vi "FormProductsTable.vi"() -> ()   [LabVIEW 2012]
uses:
  resultShow.vi
  S7Ref.vi
panel:
  in  "检具选择":bool[](array[boolean])
  in  "判定设定 2":string[][](table)
  in  "参数设定 2":string[][](table)
  in  "判定设定":string[][](table)
  in  "参数设定":string[][](table)
  in  "产品选择":bool
  in  "产品删除":bool
  in  "产品更新":bool
  in  "产品注册":bool
  in  "产品":string(combo)
  # "检具15"
  # "检具1"
  # "检具2"
  # "检具3"
  # "检具4"
  # "检具5"
  # "检具6"
  # "检具7"
  # "检具8"
  # "检具9"
  # "检具10"
  # "检具11"
  # "检具12"
  # "检具13"
  # "检具14"
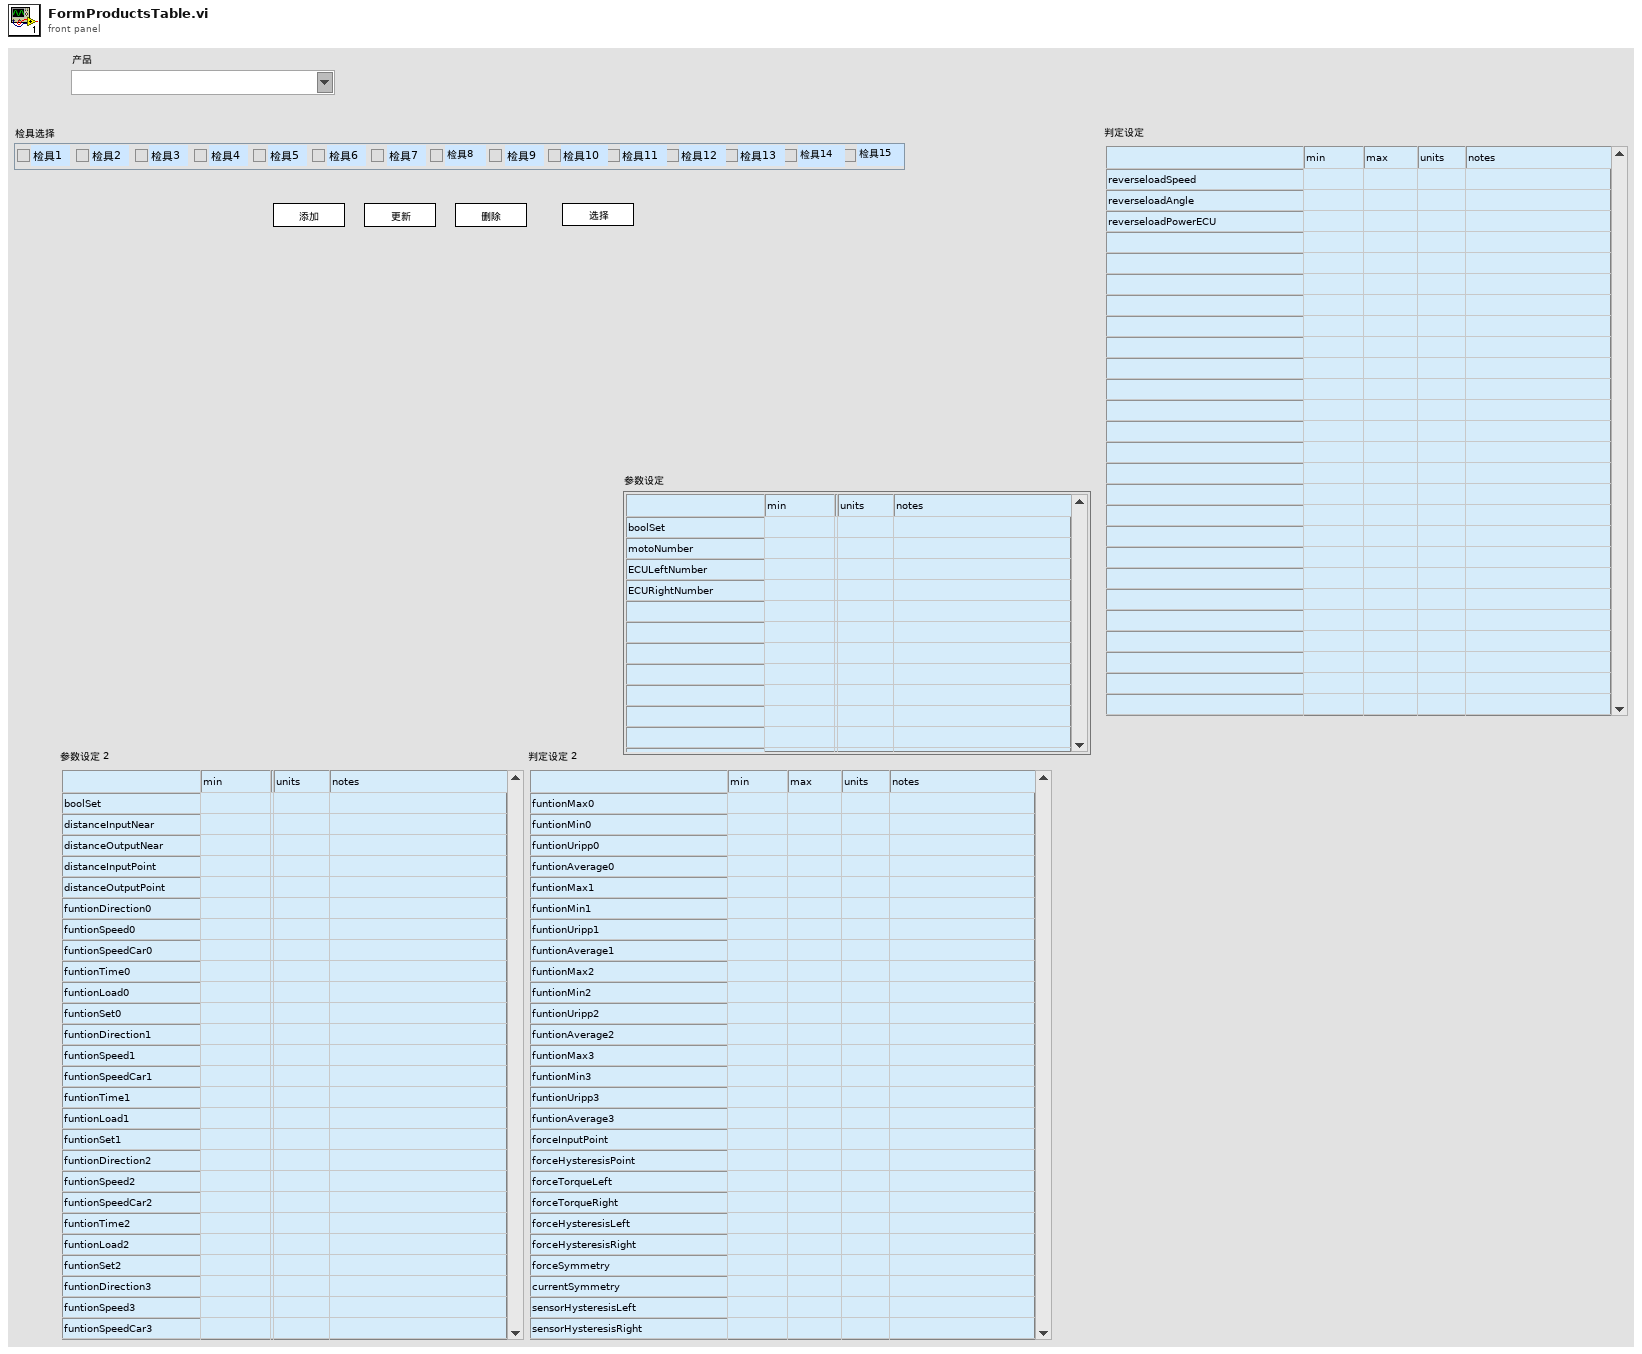
[diagram p1: front panel]
types:
  T1 = enum8{"Enabled", "Disabled", "Disabled and Grayed Out"}
  T2 = enum16{"selectdata", "selectsave", "selectlist", "selectshow"}
  T3 = cluster{"userCode":string, "userName":string, "userStatus":string, "connectionMode":string, "takesTime":string, "countDone":string, "countOK":string, "countNG":string, "rigStatus":string, "productsName":string, "partCode1":string, "partCode2":string, "partCode3":string}
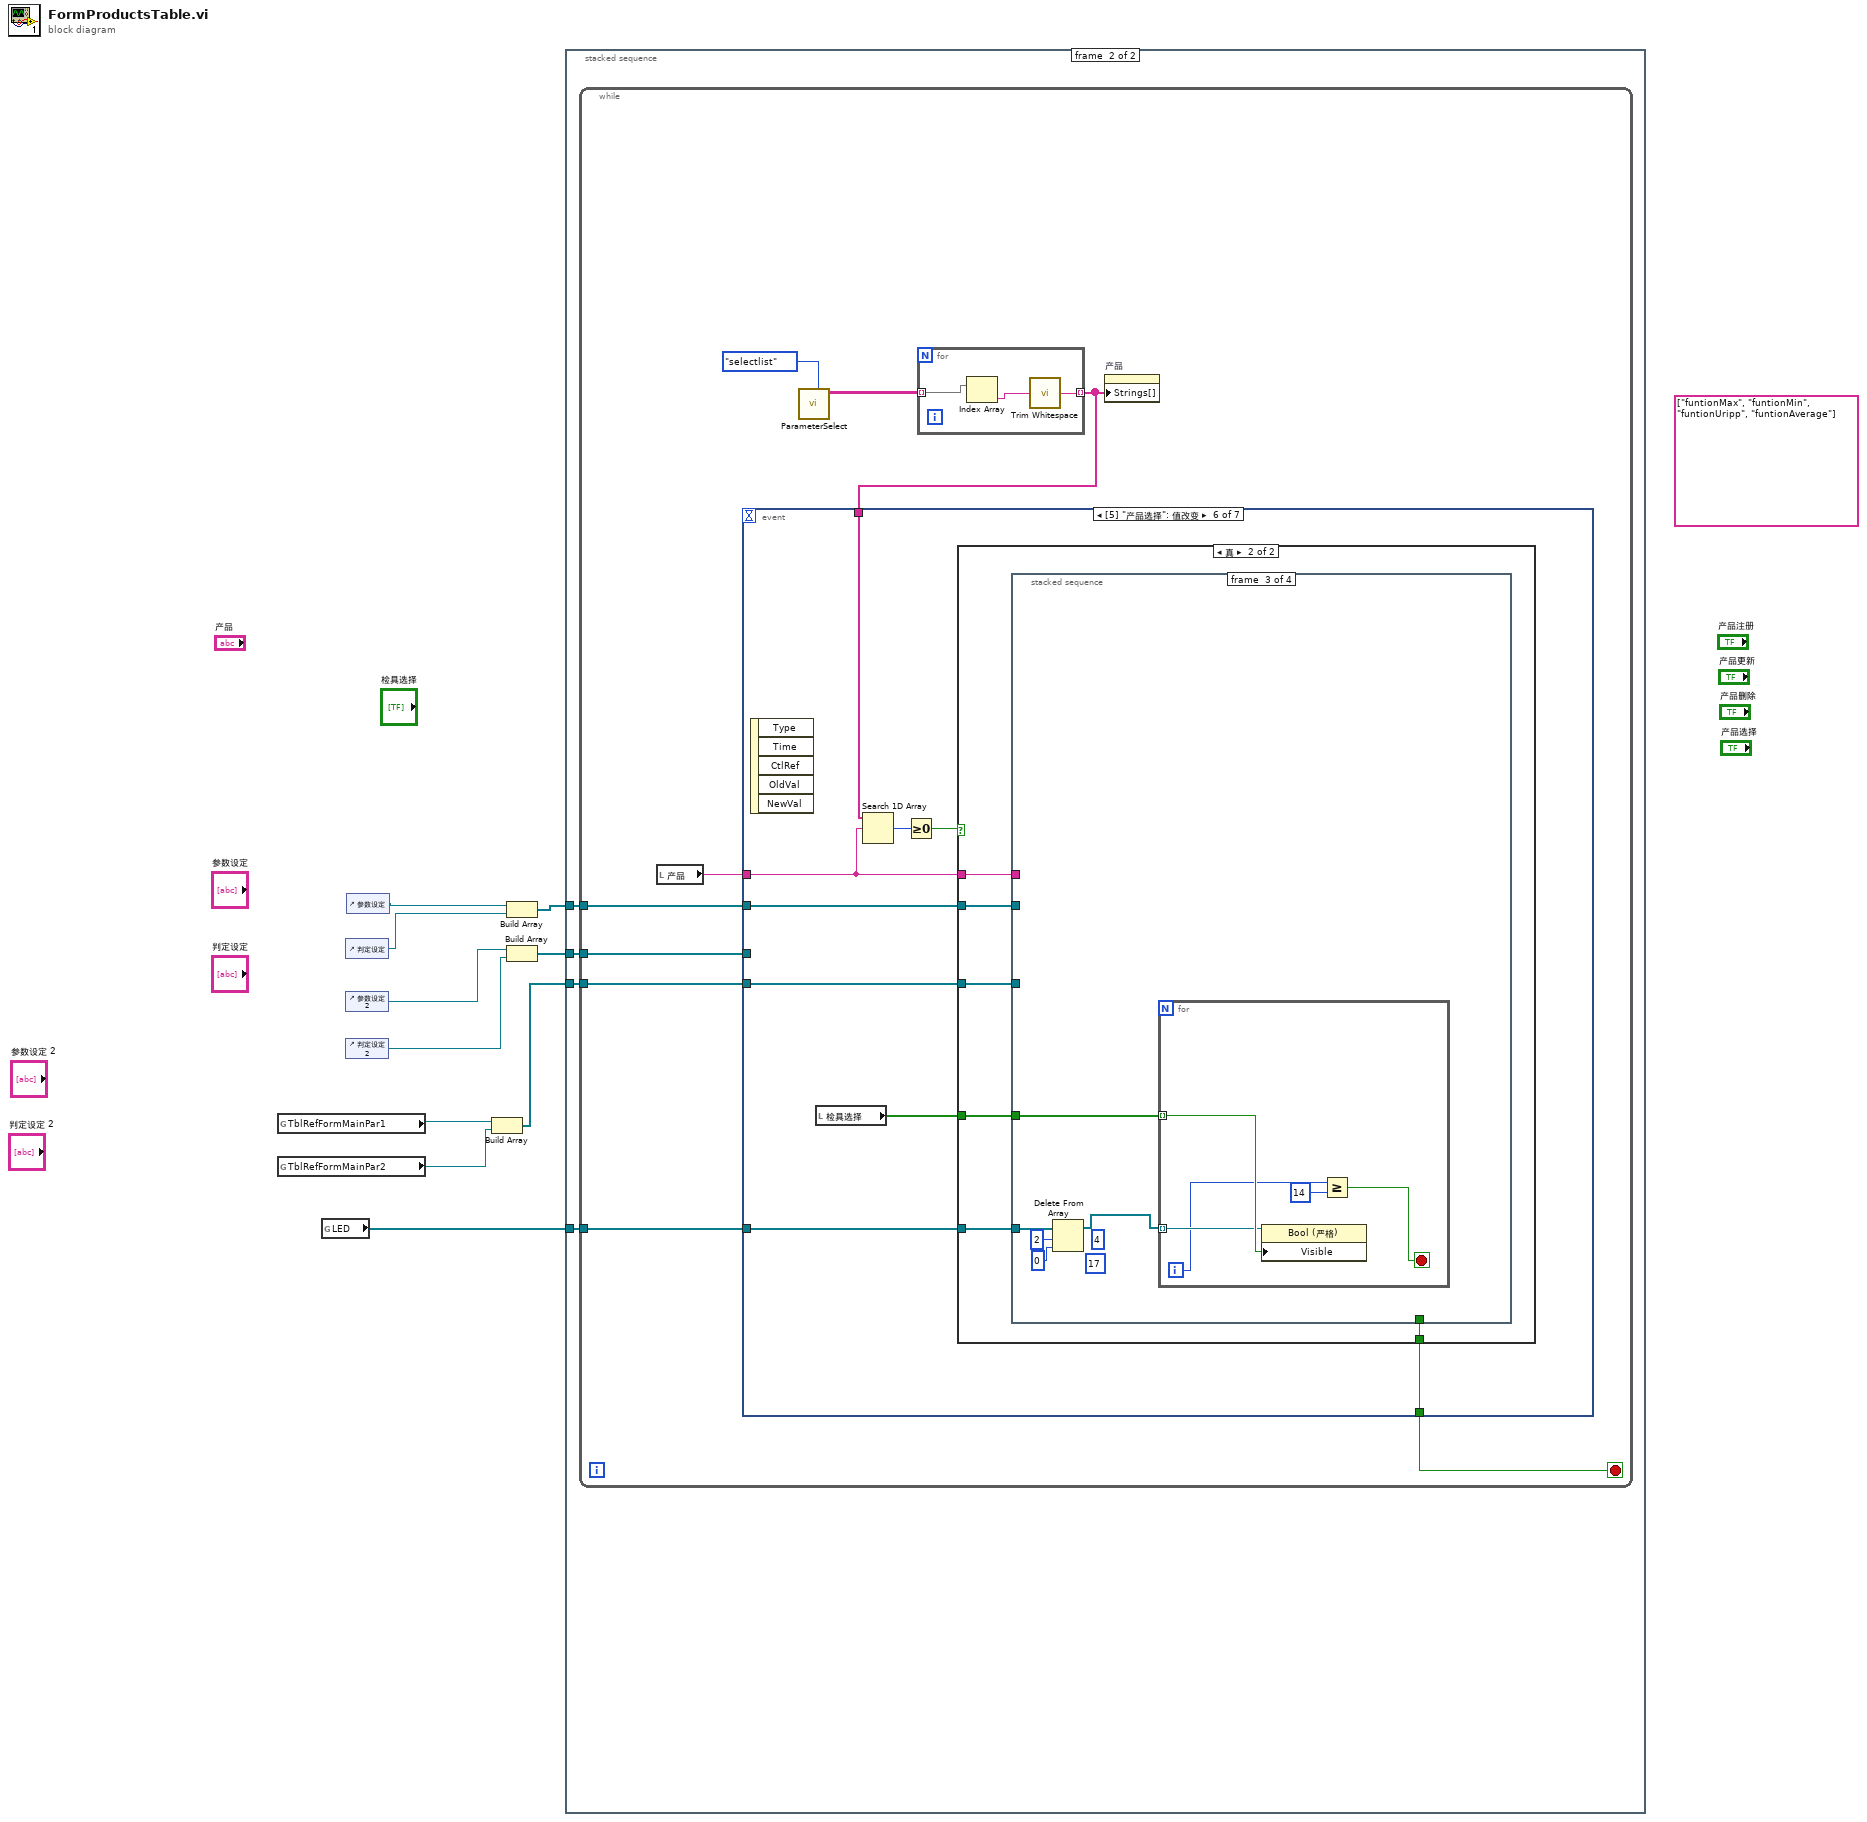
[diagram p0: block diagram]
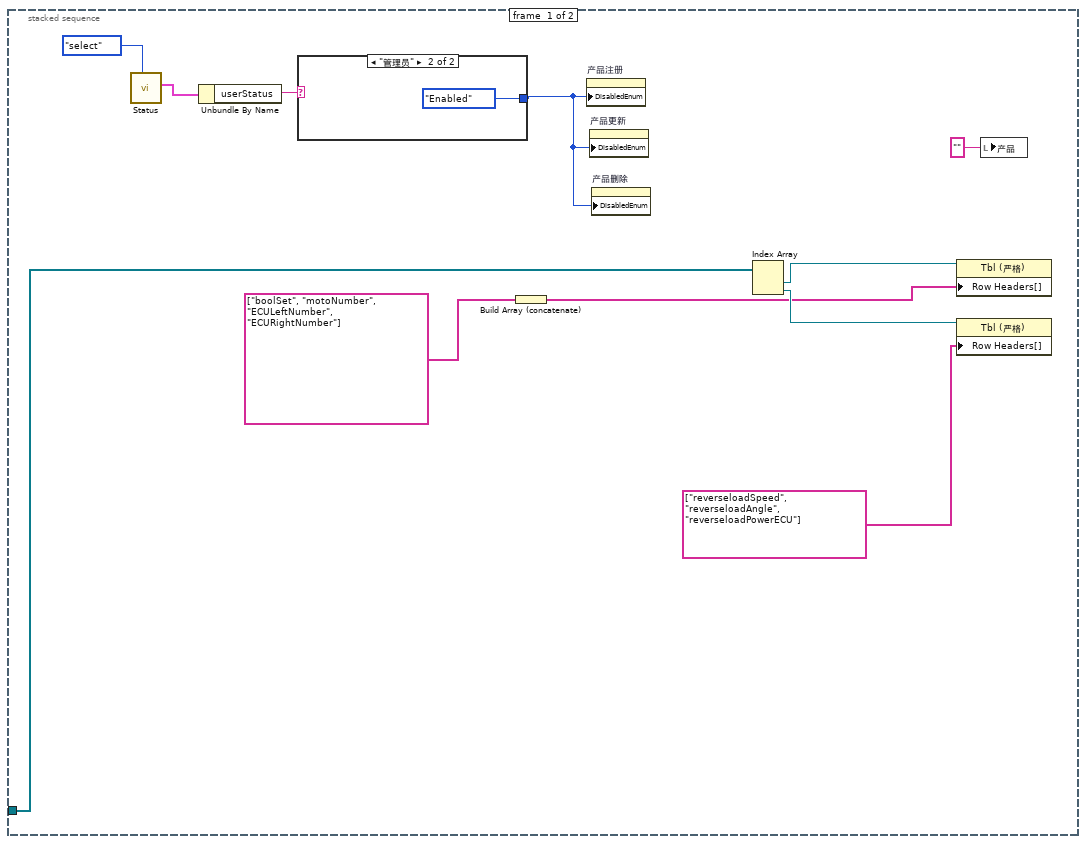
[diagram p2: hidden frame]
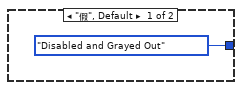
[diagram p3: hidden frame]
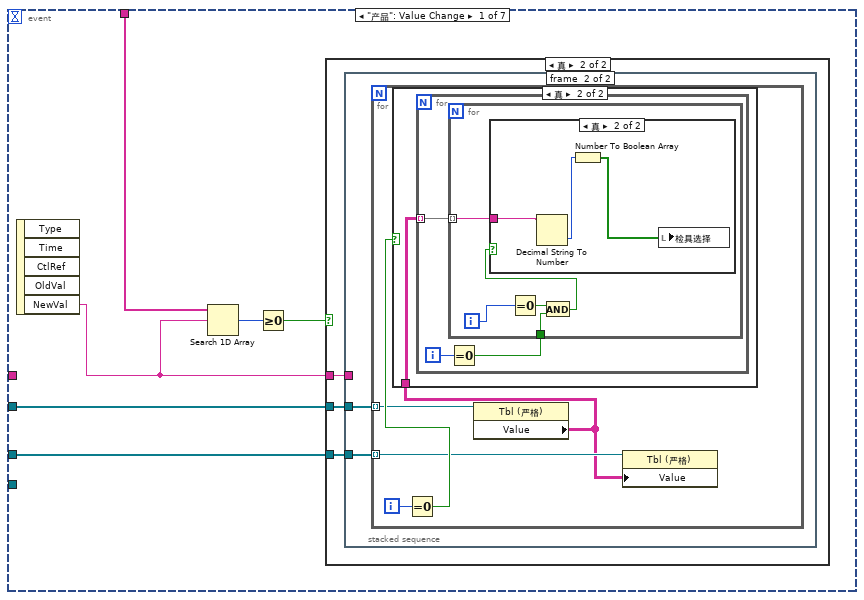
[diagram p4: hidden frame]
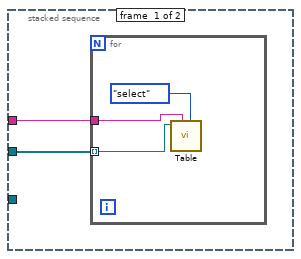
[diagram p6: hidden frame]
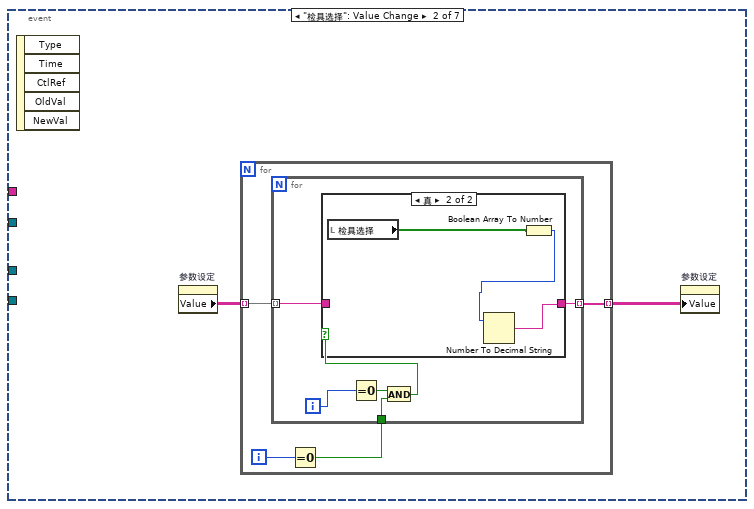
[diagram p9: hidden frame]
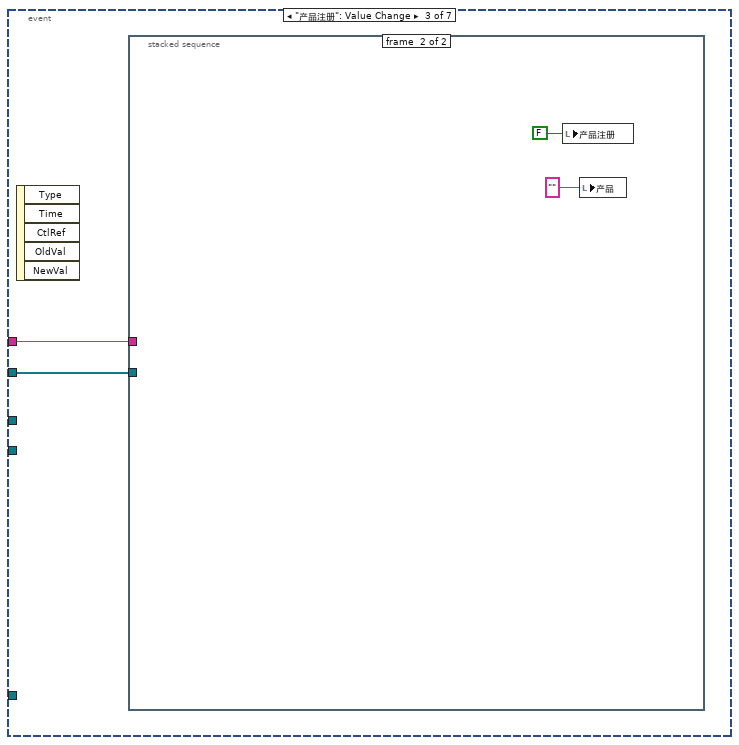
[diagram p11: hidden frame]
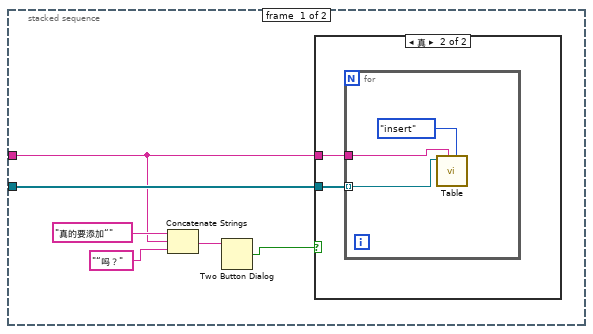
[diagram p12: hidden frame]
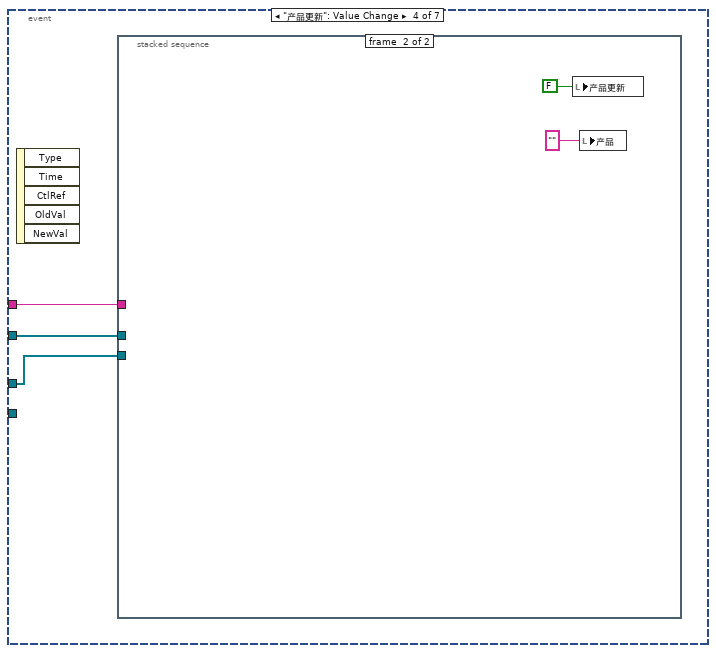
[diagram p14: hidden frame]
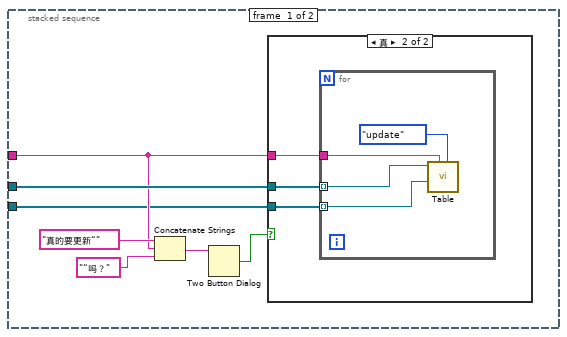
[diagram p15: hidden frame]
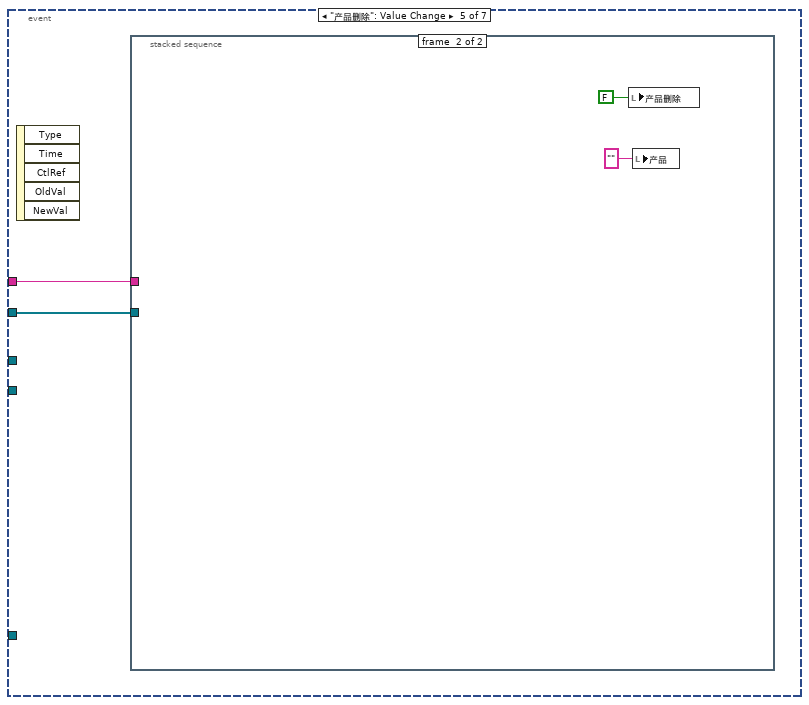
[diagram p17: hidden frame]
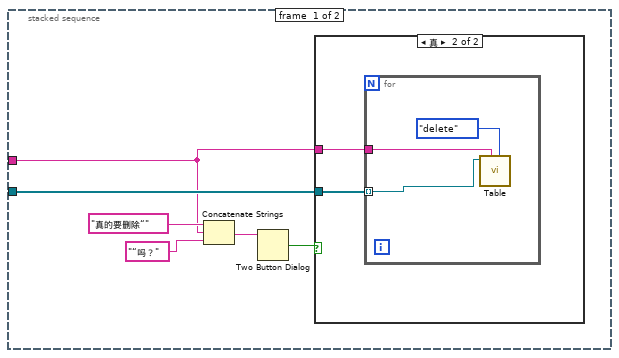
[diagram p18: hidden frame]
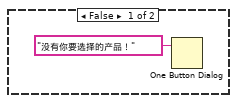
[diagram p20: hidden frame]
diagram:
  (unwired) string[] ["funtionMax", "funtionMin", "funtionUripp", "funtionAverage"] ("字符串[]")
  n1 = global read "resultShow.vi" "TblRefFormMainPar1"() -> (w6:refnum<vi>)
  n2 = global read "resultShow.vi" "TblRefFormMainPar2"() -> (w5:refnum<vi>)
  n3 = global read "resultShow.vi" "LED"() -> (w1:refnum<vi>[])
  n4 = control-ref of="判定设定"() -> (w8:refnum<vi>)
  n5 = control-ref of="参数设定 2"() -> (w3:refnum<vi>)
  n6 = control-ref of="判定设定 2"() -> (w4:refnum<vi>)
  n7 = control-ref of="参数设定"() -> (w9:refnum<vi>)
  n8 = Build Array(w6, w5) -> (w7:refnum<vi>[])
  n9 = Build Array(w9, w8) -> (w10:refnum<vi>[])
  n10 = Build Array(w3, w4) -> (w2:refnum<vi>[])
  n11 = stacked-sequence {
    tunnel: w10 -> [w14 w27]
    tunnel: w7 -> [_ w26]
    tunnel: w2 -> [_ w25]
    tunnel: w1 -> [_ w24]
    frame #0 {
      n12 = call "Status.vi"("模式"=enum16{"select", "insert", "update", "delete"}."select") -> ("元素"=w18:T3)  [unwired: 10 in]
      n13 = Unbundle By Name(w18) -> ("userStatus"=w20:string)
      n14 = case shown="\"管理员\"" w20 {
        tunnel: [T1."Disabled and Grayed Out" ("禁用") T1."Enabled" ("禁用")] -> w17
        frame "假", Default {
        }
        frame "管理员" {
        }
      }
      n15 = Build Array (concatenate)(string[] ["boolSet", "motoNumber", "ECULeftNumber", "ECURightNumber"] ("字符串[]")) -> (w13:string[])
      n16 = property on="产品注册" class="Bool (严格)"("DisabledEnum"=w17) -> ()  [unwired: 2 in, 2 out]
      n17 = property on="产品更新" class="Bool (严格)"("DisabledEnum"=w17) -> ()  [unwired: 2 in, 2 out]
      n18 = property on="产品删除" class="Bool (严格)"("DisabledEnum"=w17) -> ()  [unwired: 2 in, 2 out]
      n19 = Index Array(array=w14) -> (element #1=w16:refnum<vi>, element #2=w15:refnum<vi>)  [unwired: 2 in]
      n20 = property class="Tbl (严格)"(reference=w16, "Row Headers[]"=w13) -> ()  [unwired: 1 in, 2 out]
      n21 = property class="Tbl (严格)"(reference=w15, "Row Headers[]"=string[] ["reverseloadSpeed", "reverseloadAngle", "reverseloadPowerECU"] ("字符串[]")) -> ()  [unwired: 1 in, 2 out]
      n22 = local write "产品"("" ("y")) -> ()
    }
    frame #1 {
      n23 = while {
        tunnel: w27 -> [w33]
        tunnel: w26 -> [w30]
        tunnel: w25 -> [w29]
        tunnel: w24 -> [w28]
        stop <- w36 stop-if-true
        n24 = local read "产品"() -> (w35:string)
        n25 = call "ParameterSelect.vi"("模式"=T2."selectlist") -> ("dataOutAll"=w32:string[][])  [unwired: 5 in, 5 out]
        n26 = for {
          tunnel: w32 -> [w38] mode=indexing
          tunnel: [w39] -> w34 mode=indexing
          n27 = Index Array(array=w38) -> (element=w37:string)  [unwired: 1 in]
          n28 = call <vilib>:"Trim Whitespace.vi"("string"=w37) -> ("trimmed string"=w39:string)  [unwired: 1 in]
        }
        n29 = event shown="[5] \"产品选择\": 值改变" {
          selector: _ -> [_ _ _ _ _ _ _]
          dyn-events: _ -> [_ _ _ _ _ _ _]
          timeout: _ -> [_ _ _ _ _ _ _]
          tunnel: [_ _ _ _ _ w146 w204] -> w36
          tunnel: w33 -> [w45 _ w90 w106 w124 w141 _]
          tunnel: w35 -> [_ _ w89 w105 w123 w144 _]
          tunnel: w34 -> [w44 _ _ _ _ w145 _]
          tunnel: w30 -> [_ _ _ _ _ w140 _]
          tunnel: w29 -> [w40 _ _ w104 _ _ _]
          tunnel: w28 -> [_ _ _ _ _ w139 _]
          event "产品": Value Change {
            n30 = event-data() -> ("NewVal"=w42:string)  [unwired: 1 in, 4 out]
            n31 = Search 1D Array(1D array=w44, element=w42) -> (index of element=w43:i32)  [unwired: 1 in]
            n32 = Greater Or Equal To 0?(x=w43) -> (x >= 0?=w41:bool)
            n33 = case shown="真" w41 {
              tunnel: w45 -> [_ w48]
              tunnel: w42 -> [_ w47]
              tunnel: w40 -> [_ w46]
              frame False {
              }
              frame True {
                n34 = stacked-sequence {
                  tunnel: w48 -> [w50 w55]
                  tunnel: w47 -> [w49 _]
                  tunnel: w46 -> [_ w54]
                  frame #0 {
                    n35 = for {
                      tunnel: w50 -> [w53] mode=indexing
                      tunnel: w49 -> [w52]
                      n36 = call "Table.vi"("模式"=enum16{"select", "insert", "update", "delete"}."select", "productsName"=w52, "Table"=w53) -> ()  [unwired: 9 in]
                    }
                  }
                  frame #1 {
                    n37 = for {
                      tunnel: w55 -> [w58] mode=indexing
                      tunnel: w54 -> [w57] mode=indexing
                      i -> [w59]
                      n38 = Equal To 0?(x=w59) -> (x = 0?=w60:bool)
                      n39 = property on="属性节点" class="Tbl (严格)"(reference=w58) -> ("Value"=w56:string[][])  [unwired: 1 in, 2 out]
                      n40 = case shown="真" w60 {
                        tunnel: w56 -> [_ w61]
                        frame False {
                        }
                        frame True {
                          n41 = for {
                            tunnel: w61 -> [w62] mode=indexing
                            i -> [w64]
                            n42 = Equal To 0?(x=w64) -> (x = 0?=w63:bool)
                            n43 = for {
                              tunnel: w62 -> [w66] mode=indexing
                              tunnel: w63 -> [w67]
                              i -> [w68]
                              n44 = Equal To 0?(x=w68) -> (x = 0?=w69:bool)
                              n45 = And(x=w69, y=w67) -> (x .and. y?=w65:bool)
                              n46 = case shown="真" w65 {
                                tunnel: w66 -> [_ w72]
                                frame False {
                                }
                                frame True {
                                n47 = Decimal String To Number(string=w72) -> (number=w71:i32)  [unwired: 2 in, 1 out]
                                n48 = Number To Boolean Array(number=w71) -> (Boolean array=w70:bool[])
                                n49 = local write "检具选择"(w70) -> ()
                                }
                              }
                            }
                          }
                        }
                      }
                      n50 = property on="属性节点" class="Tbl (严格)"(reference=w57, "Value"=w56) -> ()  [unwired: 1 in, 2 out]
                    }
                  }
                }
              }
            }
          }
          event "检具选择": Value Change {
            n51 = event-data() -> ()  [unwired: 1 in, 5 out]
            n52 = property on="参数设定" class="Tbl (严格)"() -> ("Value"=w74:string[][])  [unwired: 2 in, 2 out]
            n53 = for {
              tunnel: w74 -> [w78] mode=indexing
              tunnel: [w75] -> w73 mode=indexing
              i -> [w77]
              n54 = Equal To 0?(x=w77) -> (x = 0?=w76:bool)
              n55 = for {
                tunnel: w78 -> [w80] mode=indexing
                tunnel: w76 -> [w82]
                tunnel: [w81] -> w75 mode=indexing
                i -> [w83]
                n56 = Equal To 0?(x=w83) -> (x = 0?=w84:bool)
                n57 = And(x=w84, y=w82) -> (x .and. y?=w79:bool)
                n58 = case shown="真" w79 {
                  tunnel: [w85 w87] -> w81
                  tunnel: w80 -> [w85 _]
                  frame False {
                  }
                  frame True {
                    n59 = local read "检具选择"() -> (w86:bool[])
                    n60 = Boolean Array To Number(Boolean array=w86) -> (number=w88:u32)
                    n61 = Number To Decimal String(number=w88) -> (decimal integer string=w87:string)  [unwired: 1 in]
                  }
                }
              }
            }
            n62 = property on="参数设定" class="Tbl (严格)"("Value"=w73) -> ()  [unwired: 2 in, 2 out]
          }
          event "产品注册": Value Change {
            n63 = event-data() -> ()  [unwired: 1 in, 5 out]
            n64 = stacked-sequence {
              tunnel: w90 -> [w96 _]
              tunnel: w89 -> [w91 _]
              frame #0 {
                n65 = Concatenate Strings("真的要添加“" ("消息"), w91, "“吗？" ("消息")) -> (w93:string)
                n66 = Two Button Dialog(message=w93) -> (T button?=w92:bool)  [unwired: 2 in]
                n67 = case shown="真" w92 {
                  tunnel: w96 -> [_ w98]
                  tunnel: w91 -> [_ w97]
                  frame False {
                  }
                  frame True {
                    n68 = for {
                      tunnel: w98 -> [w100] mode=indexing
                      tunnel: w97 -> [w99]
                      n69 = call "Table.vi"("模式"=enum16{"select", "insert", "update", "delete"}."insert", "productsName"=w99, "Table"=w100) -> ()  [unwired: 9 in]
                    }
                  }
                }
              }
              frame #1 {
                n70 = local write "产品注册"(FALSE ("产品注册")) -> ()
                n71 = local write "产品"("") -> ()
              }
            }
          }
          event "产品更新": Value Change {
            n72 = event-data() -> ()  [unwired: 1 in, 5 out]
            n73 = stacked-sequence {
              tunnel: w106 -> [w113 _]
              tunnel: w105 -> [w108 _]
              tunnel: w104 -> [w107 _]
              frame #0 {
                n74 = Concatenate Strings("真的要更新“" ("消息"), w108, "“吗？" ("消息")) -> (w110:string)
                n75 = Two Button Dialog(message=w110) -> (T button?=w109:bool)  [unwired: 2 in]
                n76 = case shown="真" w109 {
                  tunnel: w113 -> [_ w116]
                  tunnel: w108 -> [_ w115]
                  tunnel: w107 -> [_ w114]
                  frame False {
                  }
                  frame True {
                    n77 = for {
                      tunnel: w116 -> [w119] mode=indexing
                      tunnel: w115 -> [w118]
                      tunnel: w114 -> [w117] mode=indexing
                      n78 = call "Table.vi"("模式"=enum16{"select", "insert", "update", "delete"}."update", "productsName"=w118, "Table 2"=w117, "Table"=w119) -> ()  [unwired: 8 in]
                    }
                  }
                }
              }
              frame #1 {
                n79 = local write "产品更新"(FALSE ("产品注册")) -> ()
                n80 = local write "产品"("") -> ()
              }
            }
          }
          event "产品删除": Value Change {
            n81 = event-data() -> ()  [unwired: 1 in, 5 out]
            n82 = stacked-sequence {
              tunnel: w124 -> [w130 _]
              tunnel: w123 -> [w125 _]
              frame #0 {
                n83 = Concatenate Strings("真的要删除“" ("消息"), w125, "“吗？" ("消息")) -> (w127:string)
                n84 = Two Button Dialog(message=w127) -> (T button?=w126:bool)  [unwired: 2 in]
                n85 = case shown="真" w126 {
                  tunnel: w130 -> [_ w132]
                  tunnel: w125 -> [_ w131]
                  frame False {
                  }
                  frame True {
                    n86 = for {
                      tunnel: w132 -> [w134] mode=indexing
                      tunnel: w131 -> [w133]
                      n87 = call "Table.vi"("模式"=enum16{"select", "insert", "update", "delete"}."delete", "productsName"=w133, "Table"=w134) -> ()  [unwired: 9 in]
                    }
                  }
                }
              }
              frame #1 {
                n88 = local write "产品删除"(FALSE ("产品删除")) -> ()
                n89 = local write "产品"("" ("products_name_in")) -> ()
              }
            }
          }
          event "产品选择": Value Change {
            n90 = event-data() -> ()  [unwired: 1 in, 5 out]
            n91 = local read "检具选择"() -> (w138:bool[])
            n92 = Search 1D Array(1D array=w145, element=w144) -> (index of element=w143:i32)  [unwired: 1 in]
            n93 = Greater Or Equal To 0?(x=w143) -> (x >= 0?=w142:bool)
            n94 = case shown="真" w142 {
              tunnel: [_ w153] -> w146
              tunnel: w144 -> [_ w152]
              tunnel: w141 -> [_ w151]
              tunnel: w140 -> [_ w150]
              tunnel: w139 -> [_ w149]
              tunnel: w138 -> [_ w148]
              frame False {
                n95 = One Button Dialog(message="没有你要选择的产品！" ("消息")) -> ()  [unwired: 1 in, 1 out]
              }
              frame True {
                n96 = stacked-sequence {
                  tunnel: w152 -> [w163 _ _ _]
                  tunnel: [_ _ _ TRUE ("产品删除")] -> w153
                  tunnel: w151 -> [w156 _ _ _]
                  tunnel: w150 -> [w157 _ _ _]
                  tunnel: w149 -> [_ w185 w191 _]
                  tunnel: w148 -> [_ _ w192 _]
                  frame #0 {
                    n97 = for {
                      tunnel: w157 -> [w167] mode=indexing
                      tunnel: w156 -> [w168] mode=indexing
                      tunnel: [w166] -> w155 mode=indexing
                      n98 = property on="属性节点" class="Tbl (严格)"(reference=w168) -> (reference out=w170:refnum<vi>, "Value"=w166:string[][])  [unwired: 1 in, 1 out]
                      n99 = property on="属性节点" class="Tbl (严格)"(reference=w170) -> ("Row Headers[]"=w169:string[])  [unwired: 1 in, 2 out]
                      n100 = property on="属性节点" class="Tbl"(reference=w167, "Value"=w166) -> (reference out=w171:refnum<vi>)  [unwired: 1 in, 1 out]
                      n101 = property on="属性节点" class="Tbl"(reference=w171, "Row Headers[]"=w169) -> ()  [unwired: 1 in, 2 out]
                    }
                    n102 = Bundle("name"="productsName", "产品"=w163) -> (w162:cluster{"name":string, "产品":string})  [unwired: 1 in]
                    n103 = Index Array(array=w155) -> (element=w154:string[][])  [unwired: 3 in]
                    n104 = Build Array(w162) -> (w161:cluster{"name":string, "产品":string}[])
                    n105 = Transpose 2D Array(2D array=w154) -> (transposed array=w158:string[][])
                    n106 = call "Status.vi"("模式"=enum16{"select", "insert", "update", "delete"}."update", "nameData"=w161) -> ()  [unwired: 9 in, 1 out]
                    n107 = Index Array(array=w158) -> (element=w160:string[])  [unwired: 2 in]
                    n108 = Fract/Exp String To Number(string=w160) -> (number=w159:dbl[])  [unwired: 3 in, 1 out]
                    n109 = for {
                      tunnel: w159 -> [w172] mode=indexing
                      i -> [w176]
                      w183 = u16 2 items=["byte", "word", "Dword"]  # 数据类型
                      (unwired) u32 1  # 写入地址
                      w182 = u16 100  # DB #
                      w184 = u8 132 items=["I/O (P)"=128, "Input (I)"=129, "Output (Q)"=130, "Bit Memory (M)"=131, "Data (DB)"=132, "Instance Data (DI)"=133, "Local Data (L)"=134, "Predecessor Local Data (VL)"=135]  # 寄存器类型
                      n110 = global read "S7Ref.vi" "S7Ref"() -> (w178:refnum<k5>)
                      n111 = Add(x=20 ("y"), y=w176) -> (x+y=w175:i32)
                      n112 = To Single Precision Float(number=w172) -> (single precision float=w173:sgl)
                      n113 = Multiply(x=w175, y=4) -> (x*y=w180:i32)
                      n114 = Type Cast(type=u32 0, x=w173) -> (*(type *) &x=w179:u32)
                      n115 = call "S7_Write.vi"("TCP"=w178, "寄存器类型"=w184, "DB #"=w182, "写入地址"=w180, "数据类型"=w183, "写入数据"=w179) -> ()  [unwired: 7 in, 3 out]
                    }
                  }
                  frame #1 {
                    n116 = for {
                      tunnel: w185 -> [w187] mode=indexing
                      n117 = property class="Bool (严格)"(reference=w187, "Visible"=TRUE ("可见")) -> ()  [unwired: 1 in, 2 out]
                    }
                  }
                  frame #2 {
                    (unwired) 17 ("索引")
                    (unwired) 4 ("长度")
                    n118 = Delete From Array(array=w191, length=2 ("长度"), index=0 ("索引")) -> (array with subset deleted=w188:refnum<vi>[])  [unwired: 1 out]
                    n119 = for {
                      tunnel: w188 -> [w196] mode=indexing
                      tunnel: w192 -> [w197] mode=indexing
                      i -> [w195]
                      stop <- w193 stop-if-true
                      n120 = property class="Bool (严格)"(reference=w196, "Visible"=w197) -> ()  [unwired: 1 in, 2 out]
                      n121 = Greater Or Equal?(x=w195, y=14) -> (x >= y?=w193:bool)
                    }
                  }
                  frame #3 {
                    n122 = case shown="真" TRUE {
                      frame False {
                      }
                      frame True {
                        n123 = property on="窗格" class="Pane"() -> ("OwningVI"=w203:refnum<vi>)  [unwired: 2 in, 2 out]
                        n124 = property on="属性节点" class="VI"(reference=w203) -> ("Name"=w202:string)  [unwired: 1 in, 2 out]
                        n125 = call "CloseVI.vi"("名称或相对路径"=w202) -> ()  [unwired: 10 in, 1 out]
                      }
                    }
                    n126 = local write "产品选择"(FALSE ("产品删除")) -> ()
                    n127 = local write "产品"("") -> ()
                  }
                }
              }
            }
          }
          event Panel Close? {
            w204 = TRUE
            n128 = event-data() -> ()  [unwired: 1 in, 3 out]
            n129 = Not(x=w204) -> (.not. x?=w205:bool)
            n130 = event-data("Discard?"=w205) -> ()  [unwired: 1 in, 1 out]
          }
        }
        n131 = property on="产品" class="CmbBox"("Strings[]"=w34) -> ()  [unwired: 2 in, 2 out]
      }
    }
  }
